vi "first-try.vi"() -> ()   [LabVIEW 2011]
uses:
  <vilib>/Instr/_visa.llb/VISA Configure Serial Port (Instr).vi
panel:
  out "ExecTime":u32
  out "Boolean array":bool[](array[boolean])
  out "DataCluster":T1
  in  "BaudRate":u32(ring) items=["9600"=9600, "115200"=65535]
  in  "VISA resource name":refnum<visa-resource-name>
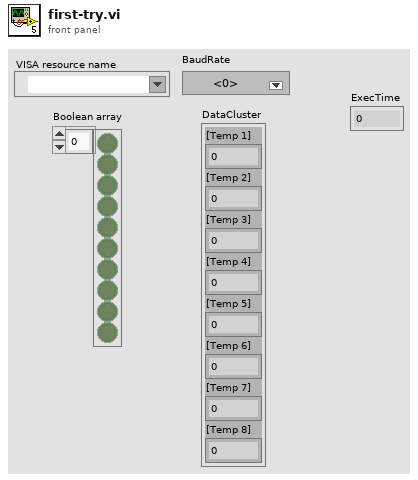
[diagram p1: front panel]
types:
  T1 = cluster{"[Temp 1]":dbl, "[Temp 2]":dbl, "[Temp 3]":dbl, "[Temp 4]":dbl, "[Temp 5]":dbl, "[Temp 6]":dbl, "[Temp 7]":dbl, "[Temp 8]":dbl}
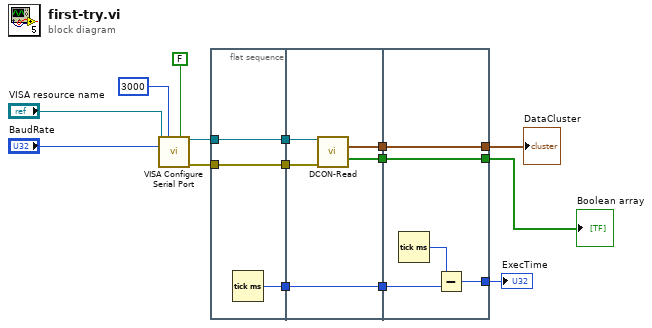
[diagram p0: block diagram]
diagram:
  n1 = call-poly "VISA Configure Serial Port"("VISA resource name"="VISA resource name", "timeout (10sec)"=u32 3000, "Enable Termination\nChar (T)"=FALSE ("Enable Termination\nChar (T)"), "baud rate (9600)"="BaudRate") -> ("VISA resource name out"=w11:refnum<visa-resource-name>, "error out"=w10:errorcluster)  [unwired: 10 in]
  n2 = flat-sequence {
    tunnel: w10 -> [w17]
    tunnel: w11 -> [w18]
    tunnel: [w18] -> w5
    tunnel: [w17] -> w4
    tunnel: [w16] -> w2
    tunnel: [w21] -> w7
    tunnel: [w20] -> w6
    tunnel: w5 -> [w23]
    tunnel: w4 -> [w22]
    tunnel: [w19] -> w3
    tunnel: w2 -> [w19]
    tunnel: [w27] -> w8
    tunnel: [w28] -> w9
    tunnel: w7 -> [w28]
    tunnel: w6 -> [w27]
    tunnel: w3 -> [w25]
    tunnel: [w24] -> w1
    frame #0 {
      n3 = Tick Count (ms)() -> (millisecond timer value=w16:u32)
    }
    frame #1 {
      n4 = call "DCON-Read.vi"("VRN in"=w23, "error in (no error)"=w22) -> ("DataCluster"=w21:T1, "Boolean array"=w20:bool[])  [unwired: 10 in, 2 out]
    }
    frame #2 {
      n5 = Tick Count (ms)() -> (millisecond timer value=w26:u32)
      n6 = Subtract(x=w26, y=w25) -> (x-y=w24:u32)
    }
  }
  "DataCluster" <- w9
  "Boolean array" <- w8
  "ExecTime" <- w1
